vi "PushTask Globals.vi"() -> ()   [LabVIEW 2017]
panel:
  in  "sample count":i32
  in  "stop all":bool
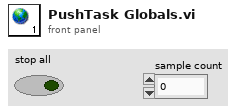
[diagram p1: front panel]
diagram:
